vi "Step_Delay_Tommaso_fixed_EPICS2.vi"() -> ()   [LabVIEW 2020]
uses:
  <vilib>/DAQmx/write.llb/DAQmx Write (Analog DBL 1Chan 1Samp).vi
  <vilib>/DAQmx/miscellaneous.llb/DAQmx Fill In Error Info.vi
  <vilib>/DAQmx/create/channels.llb/DAQmx Create Channel (AO-Voltage-Basic).vi
  <userlib>/caLab/Private/Put_Boolean-1D_PV.vi
  <userlib>/caLab/Private/Put_DBL_PV.vi
  <vilib>/Analysis/1siggen.llb/Ramp Pattern by Delta.vi
  libs/Newport ESP301/Newport ESP301.lvlib
  <vilib>/Analysis/NI_AALBase.lvlib
panel:
  in  "WP2 pos B":dbl=30.0
  in  "WP1 pos B":dbl=10.0
  in  "WP2 pos A":dbl=35.0
  in  "WP1 pos A":dbl=15.0
  out "moving":bool
  out "running":bool
  out "wp2 position [deg]":dbl=35.0 format="%.6g"
  out "wp1 position [deg]":dbl=15.0 format="%.6g"
  in  "Tab Control":enum32{"equally spaced", "user-defined"}(tab)
  in  "StepSize [fs]":i32=1000
  out "StepSize [mm]":dbl=0.14989622900000002
  in  "Wait time [ms]":u32=1000
  in  "go2p1":bool
  in  "p2 [mm]":dbl=0.1
  in  "p1 [mm]":dbl=-0.1
  in  "Delta2 [fs]":dbl=6384.750346187828
  in  "Delta1 [fs]":dbl=5050.49396539522
  in  "Dwell_positions":string[][](table)=[["5000", "3000"], ["5100", "3000"], ["5200", "5000"], ["5300", "5000"], ["5500", "5000"], ["6000", "10000"], ["", ""], ["", ""]]
  out "IOC started":bool=TRUE
  in  "Config File":path=path "T:/trARPES/Labview/Front ends/METIS_delayscan/delayScanEPICS.conf" caption="Soft IOC configuration file"
  in  "Configuration Set":T1(array[cluster])=[{"PV name"="trARPES:DelayStage:t0", "description"="Delay Stage time zero Position", "data type"="ai", "number of elements (waveform only)"=1, "element size (waveform only)"="", []}, {"PV name"="trARPES:DelayStage:p1", "description"="Delay Stage range start", "data type"="ai", "number of elements (waveform only)"=1, "element size (waveform only)"="", []}, {"PV name"="trARPES:DelayStage:p2", "description"="Delay Stage range end", "data type"="ai", "number of elements (waveform only)"=1, "element size (waveform only)"="", []}, {"PV name"="trARPES:DelayStage:Pos", "description"="Current Delay Stage position", "data type"="ai", "number of elements (waveform only)"=1, "element size (waveform only)"="", []}]
  in  "stop 2":bool
  in  "Enable?":bool=TRUE
  out "a":waveform(dbl)(graph)={"t0"=timestamp(3680562352.257453 s since 1904-01-01), "dt"=1.0, "Y"=[0.04235]}
  out "Waveform Chart":dbl(graph)=6.694
  out "x*y":dbl=6.694
  in  "physical channels":tag="Dev1/ao1"
  out "DAC error":errorcluster
  out "ESP error":errorcluster
  in  "set_vel":bool
  in  "velocity [fs/s]":dbl=66.71281903963042
  in  "vel_mm":dbl=0.01 caption="velocity [mm/s]"
  out "meas. velocity":dbl
  out "output voltage":dbl=6.694
  in  "start":bool
  out "position [mm]":dbl=0.04235
  in  "interpolate output":bool
  in  "Reference [mm]":dbl=-0.85705
  in  "Axis (1)":i32[](array[numeric])=[3, 2, 1] min=1 max=3
  in  "Serial Link (RS232)":enum16{"RS232", "USB"}(ring)
  in  "VISA resource name":refnum<visa-resource-name>="COM8"
  in  "main_close":bool
  # "Interface panel"
  # "Velocity panel"
  # "delay"
  # "wp1"
  # "wp2"
  # "Positions panel"
  # "Measurement Mode"
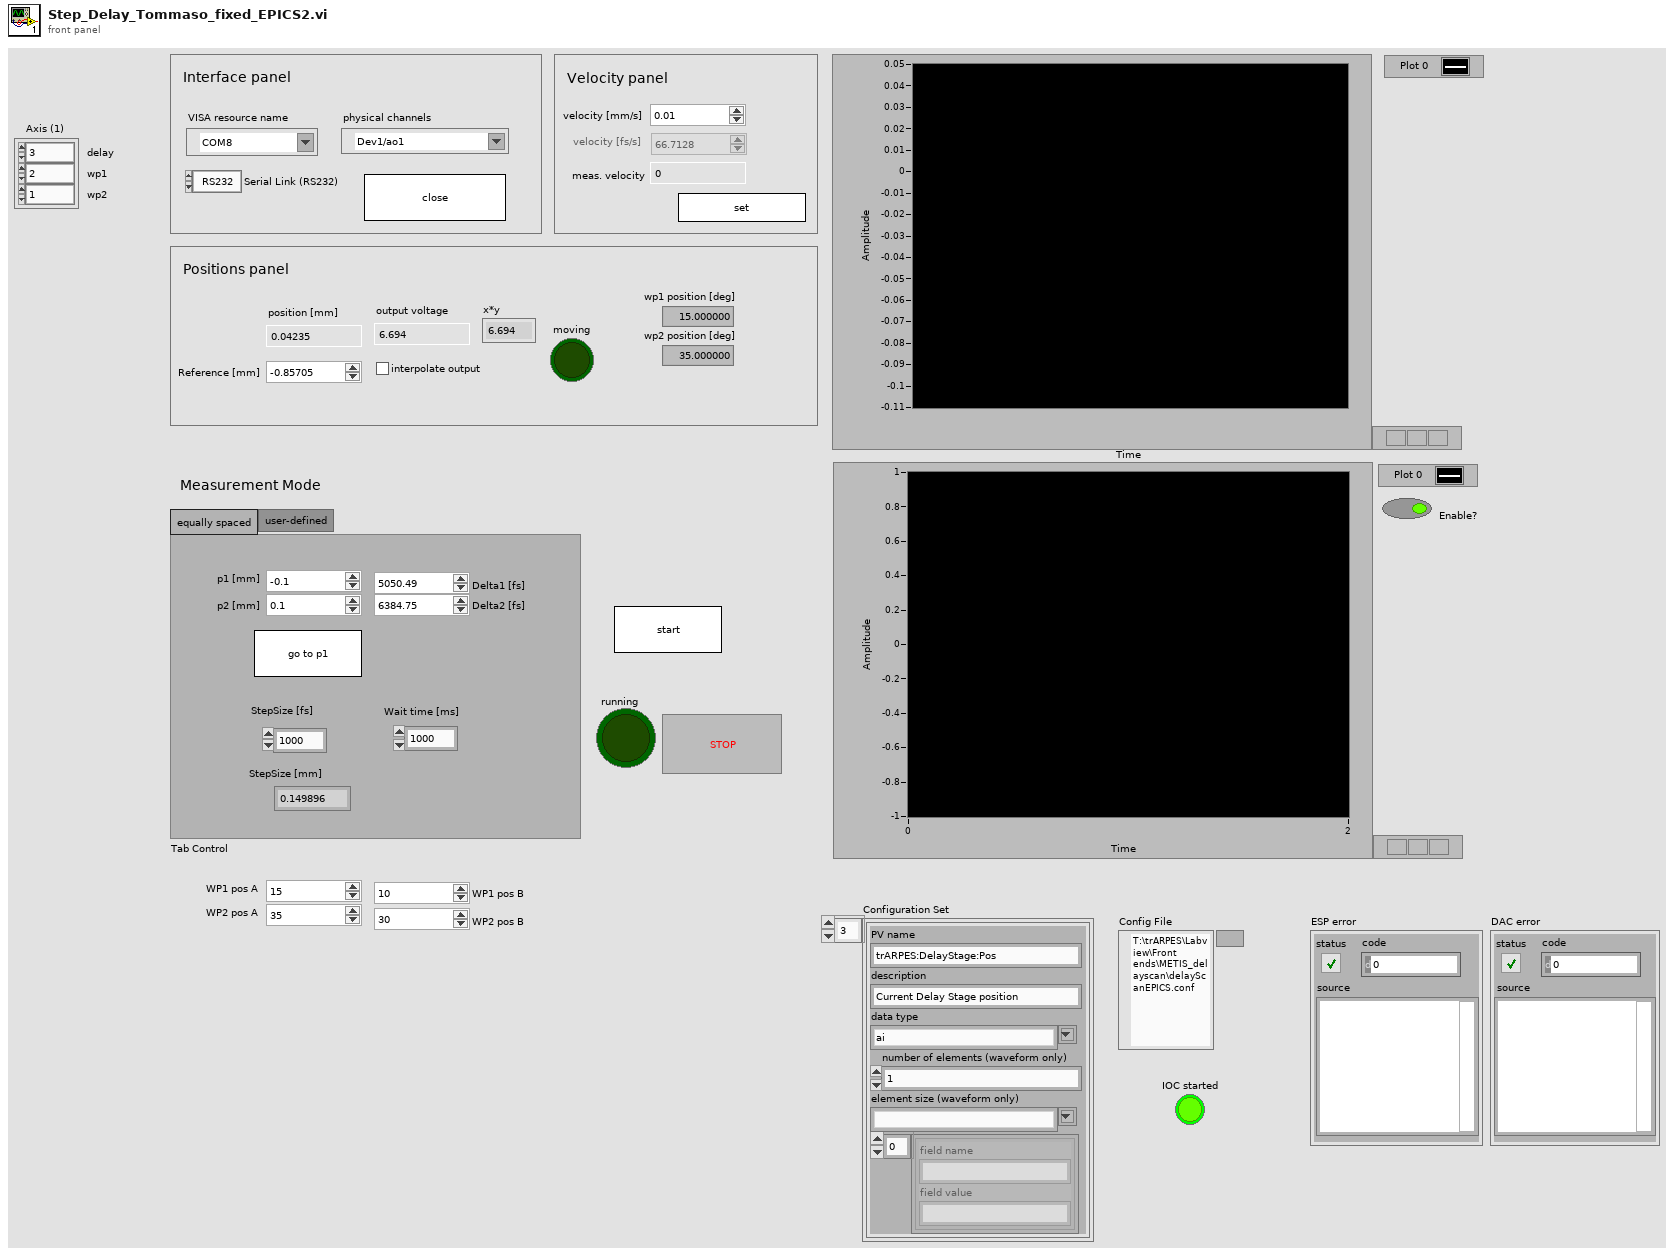
[diagram p1: front panel]
types:
  T1 = cluster{"PV name":string, "description":string, "data type":string, "number of elements (waveform only)":i32, "element size (waveform only)":string, cluster{"field name":string, "field value":string}[]}[]
  T2 = cluster{"dev1_data":refnum<queue>, "dev2_data":refnum<queue>}
  T3 = cluster{"dev1_cmd":refnum<queue>, "dev2_cmd":refnum<queue>, "meas_cmd":refnum<queue>}
  T4 = cluster{"PV Name":string, "Data Type":string, "Fields":cluster{"Field Name":string, "Field Value":string}[]}[]
  T5 = cluster{"PV Name":string, "Data Type":string, "Fields":cluster{"Field Name":string, "Field Value":string}[]}
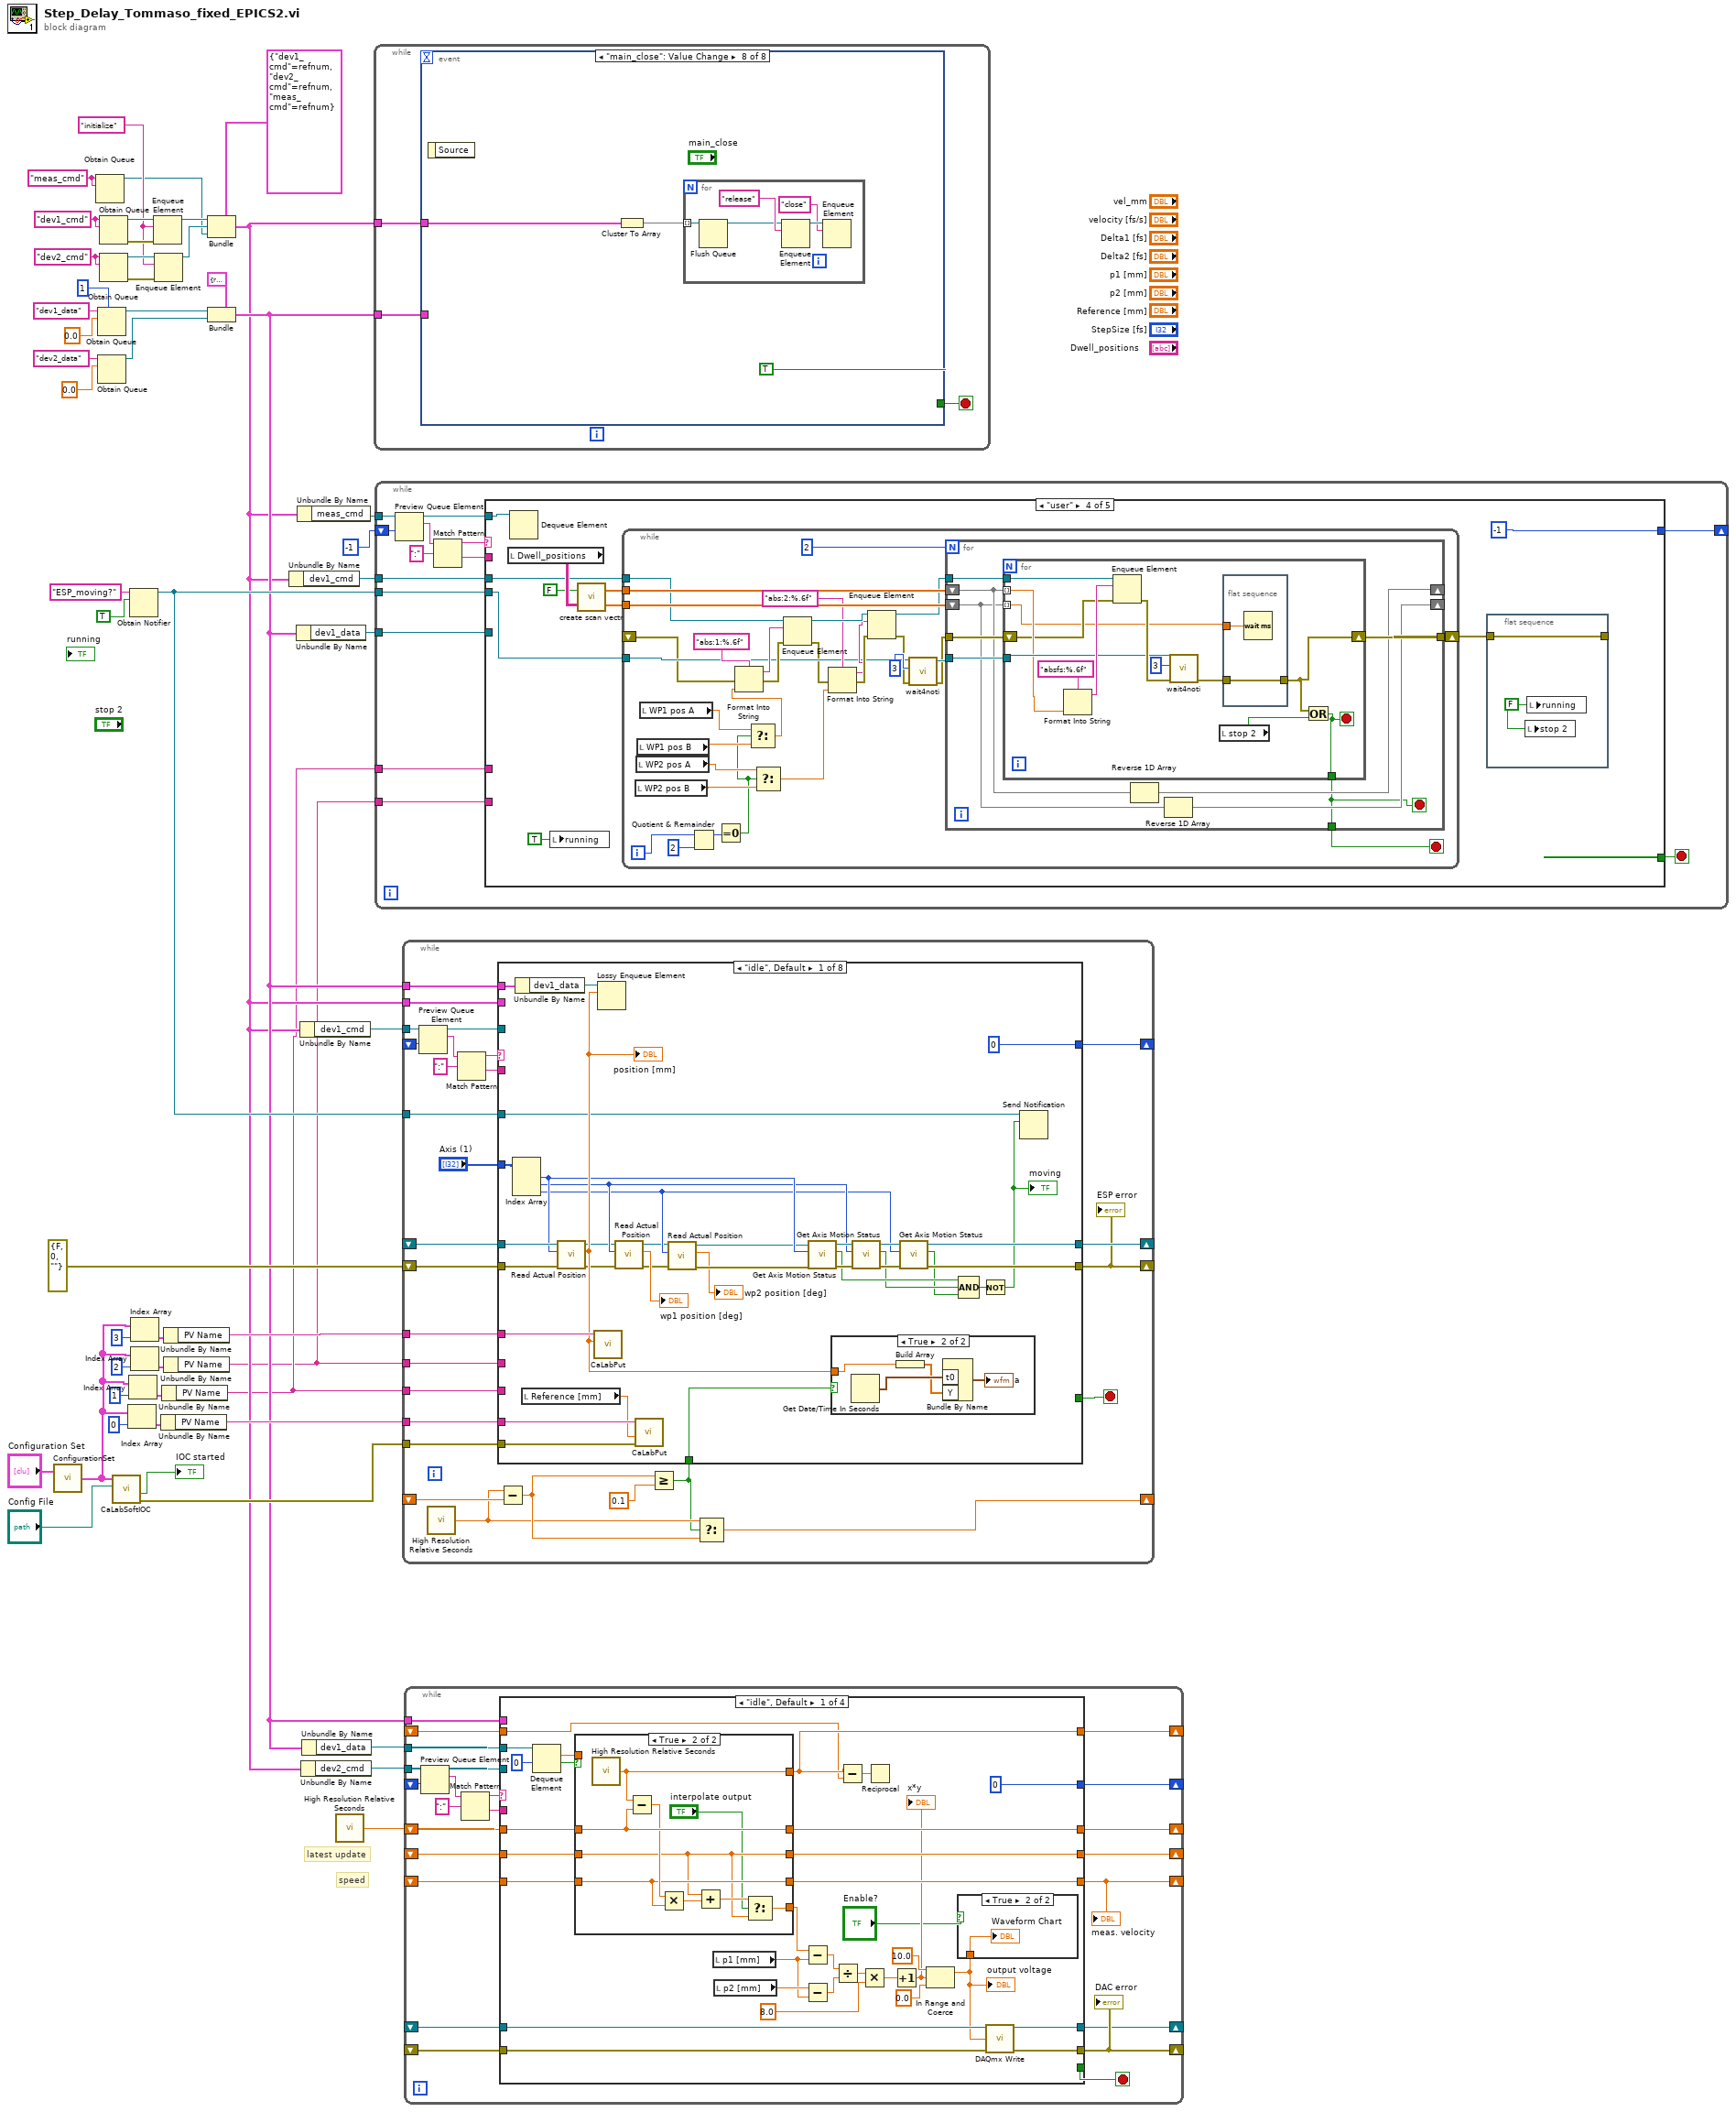
[diagram p0: block diagram]
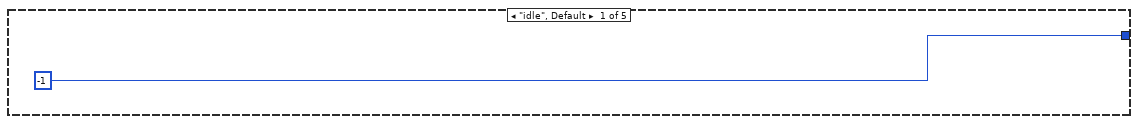
[diagram p2: hidden frame]
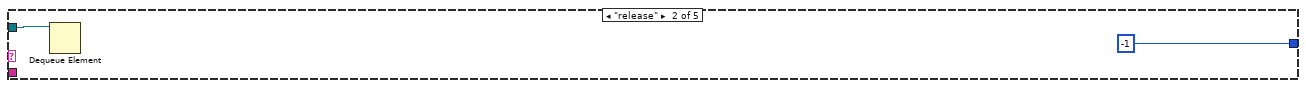
[diagram p3: hidden frame]
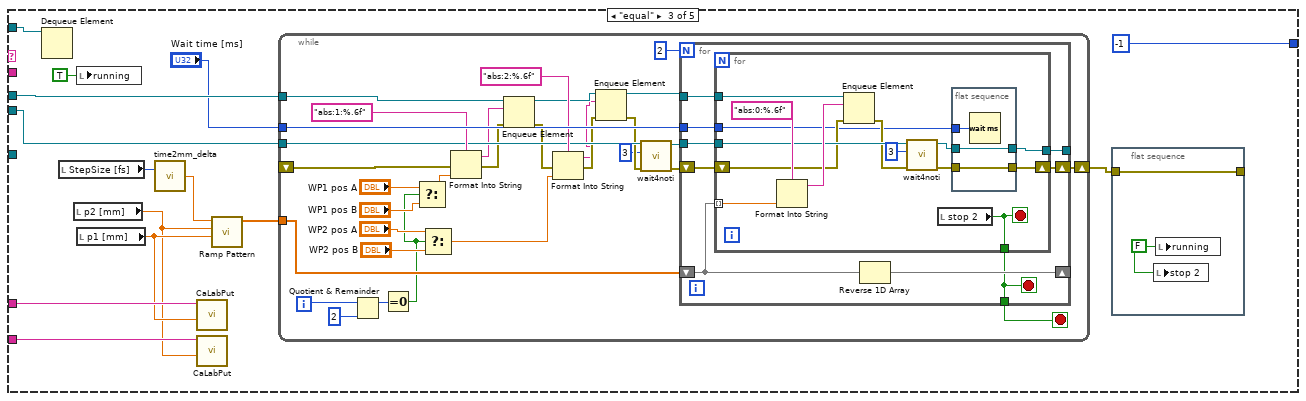
[diagram p4: hidden frame]
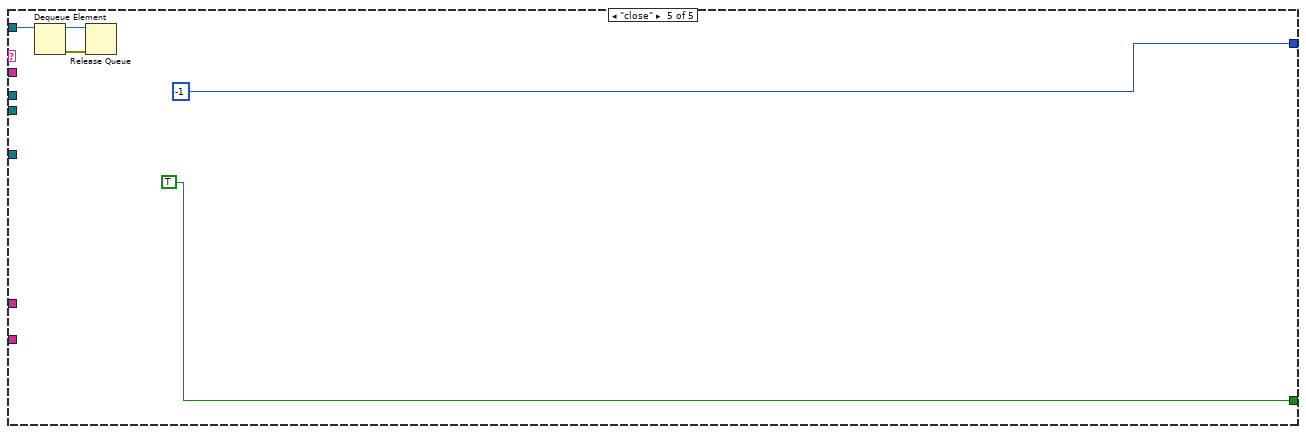
[diagram p5: hidden frame]
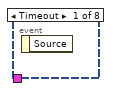
[diagram p6: hidden frame]
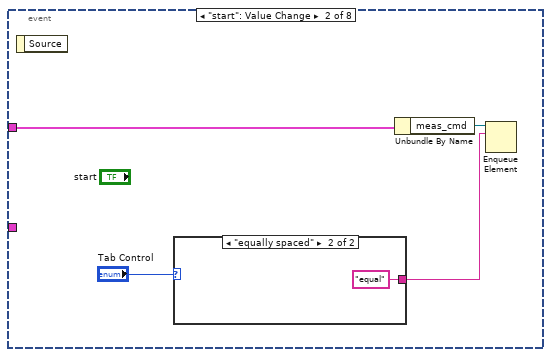
[diagram p7: hidden frame]
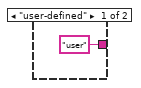
[diagram p8: hidden frame]
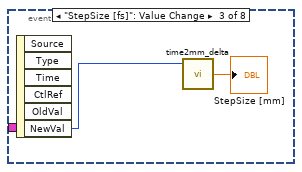
[diagram p9: hidden frame]
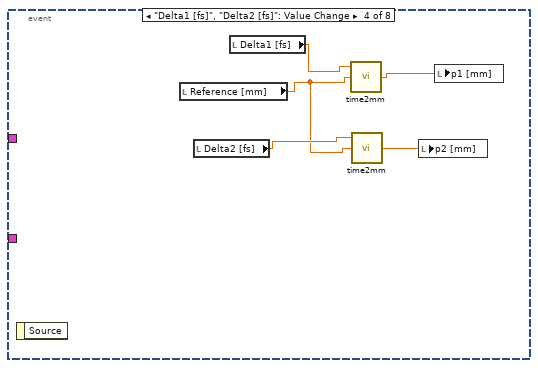
[diagram p10: hidden frame]
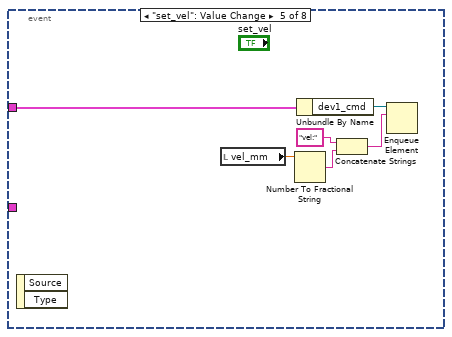
[diagram p11: hidden frame]
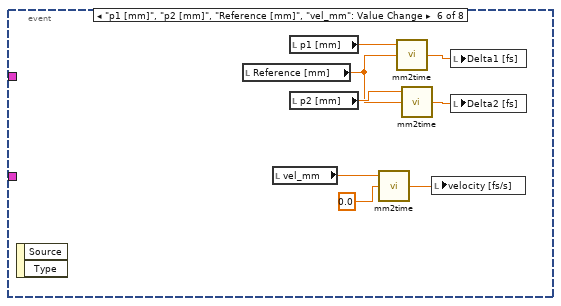
[diagram p12: hidden frame]
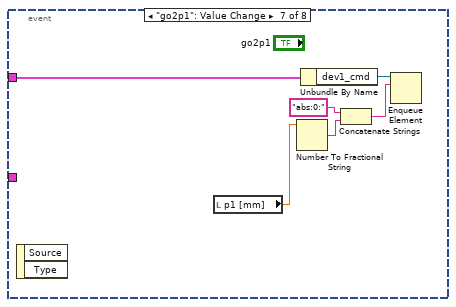
[diagram p13: hidden frame]
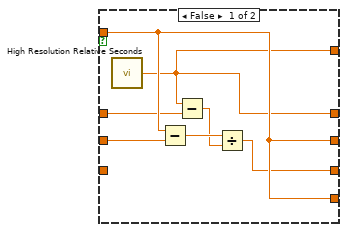
[diagram p15: hidden frame]
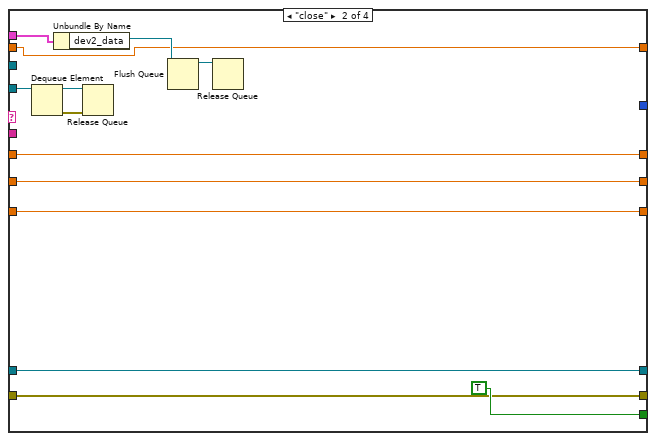
[diagram p16: hidden frame]
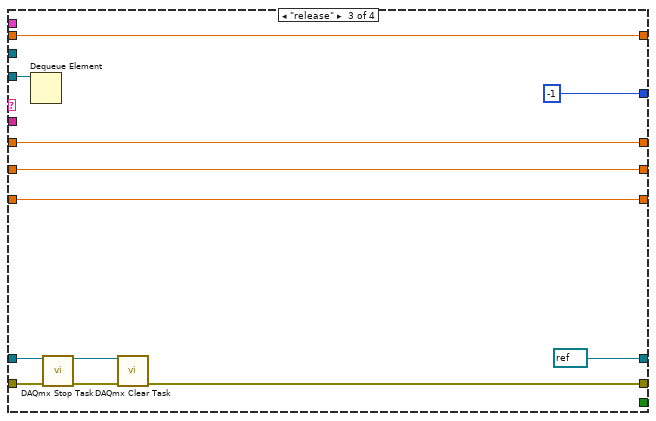
[diagram p17: hidden frame]
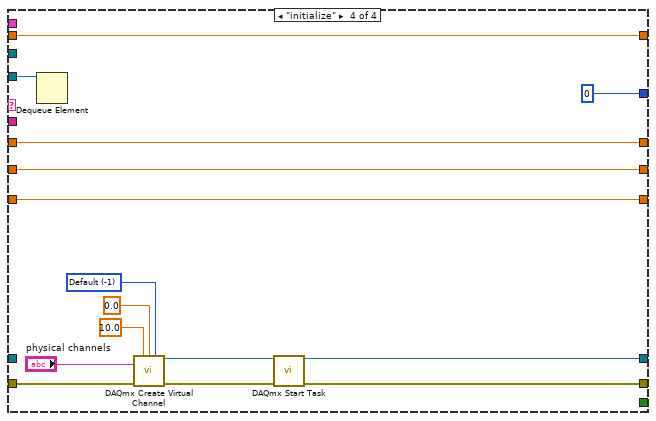
[diagram p18: hidden frame]
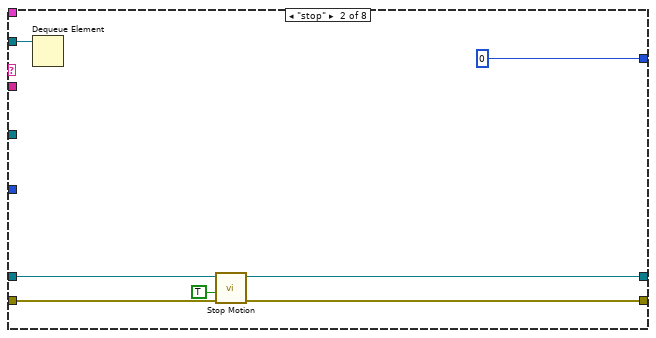
[diagram p20: hidden frame]
diagram:
  w12 = "meas_cmd" ("name (unnamed)")
  w39 = "dev2_cmd" ("name (unnamed)")
  w45 = "initialize" ("element")
  w40 = "dev1_cmd" ("name (unnamed)")
  # "speed"
  # "latest update"
  n1 = call <userlib>:"ConfigurationSet.vi"("Configuration Set"="Configuration Set") -> ("PV set"=w18:T4)  [unwired: 1 in]
  n2 = Obtain Queue(name (unnamed)=w12, element data type=w12) -> (queue out=w1:refnum<queue>)  [unwired: 3 in, 2 out]
  n3 = Obtain Queue(max queue size (-1, unlimited)=1, name (unnamed)="dev1_data", element data type=0.0) -> (queue out=w36:refnum<queue>)  [unwired: 2 in, 2 out]
  n4 = Obtain Queue(name (unnamed)="dev2_data", element data type=0.0) -> (queue out=w35:refnum<queue>)  [unwired: 3 in, 2 out]
  n5 = Obtain Queue(name (unnamed)=w40, element data type=w40) -> (queue out=w51:refnum<queue>, error out=w50:errorcluster)  [unwired: 3 in, 1 out]
  n6 = Obtain Queue(name (unnamed)=w39, element data type=w39) -> (queue out=w46:refnum<queue>, error out=w47:errorcluster)  [unwired: 3 in, 1 out]
  n7 = call <userlib>:"CaLabSoftIOC.vi"("Config File"="Config File", "PV set"=w18) -> ("error out"=w16:errorcluster, "IOC started"=→"IOC started":bool)  [unwired: 4 in, 2 out]
  n8 = Index Array(array=w18, index=0) -> (element=w27:T5)
  n9 = Index Array(array=w18, index=1) -> (element=w23:T5)
  n10 = Obtain Notifier(name (unnamed)="ESP_moving?", notification data type=TRUE) -> (notifier out=w9:refnum<notifier>)  [unwired: 2 in, 2 out]
  n11 = Index Array(array=w18, index=3) -> (element=w19:T5)
  n12 = Index Array(array=w18, index=2) -> (element=w22:T5)
  n13 = Enqueue Element(queue=w51, element=w45, error in (no error)=w50) -> (queue out=w48:refnum<queue>)  [unwired: 1 in, 2 out]
  n14 = Enqueue Element(queue=w46, element=w45, error in (no error)=w47) -> (queue out=w44:refnum<queue>)  [unwired: 1 in, 2 out]
  n15 = Unbundle By Name(w27) -> ("PV Name"=w15:string)
  n16 = Unbundle By Name(w23) -> ("PV Name"=w3:string)
  n17 = Unbundle By Name(w19) -> ("PV Name"=w14:string)
  n18 = Unbundle By Name(w22) -> ("PV Name"=w2:string)
  n19 = Bundle(cluster=T3 {"dev1_cmd"=refnum, "dev2_cmd"=refnum, "meas_cmd"=refnum}, "dev1_cmd"=w48, "dev2_cmd"=w44, "meas_cmd"=w1) -> (w5:T3)
  n20 = Bundle(cluster=T2 {"dev1_data"=refnum, "dev2_data"=refnum}, "dev1_data"=w36, "dev2_data"=w35) -> (w7:T2)
  n21 = Unbundle By Name(w5) -> ("dev1_cmd"=w4:refnum<queue>)
  n22 = Unbundle By Name(w7) -> ("dev1_data"=w6:refnum<queue>)
  n23 = Unbundle By Name(w5) -> ("meas_cmd"=w13:refnum<queue>)
  n24 = Unbundle By Name(w5) -> ("dev1_cmd"=w41:refnum<queue>)
  n25 = Unbundle By Name(w5) -> ("dev2_cmd"=w32:refnum<queue>)
  n26 = Unbundle By Name(w7) -> ("dev1_data"=w31:refnum<queue>)
  n27 = call <vilib>:"High Resolution Relative Seconds.vi"() -> ("relative seconds"=w30:dbl)
  n28 = while {
    tunnel: w5 -> [w54]
    tunnel: w7 -> [w53]
    stop <- w52 stop-if-true
    n29 = event shown="[7] \"main_close\": Value Change" {
      selector: _ -> [_ _ _ _ _ _ _ _]
      dyn-events: _ -> [_ _ _ _ _ _ _ _]
      timeout: _ -> [_ _ _ _ _ _ _ _]
      tunnel: w54 -> [_ w57 _ _ w69 _ w87 w90]
      tunnel: w53 -> [_ _ _ _ _ _ _ _]
      tunnel: [_ _ _ _ _ _ _ TRUE] -> w52
      event Timeout {
        n30 = event-data() -> ()  [unwired: 1 in, 1 out]
      }
      event "start": Value Change {
        n31 = event-data() -> ()  [unwired: 1 in, 1 out]
        n32 = case shown="\"equally spaced\"" "Tab Control" {
          tunnel: ["user" "equal"] -> w55
          frame "user-defined" {
          }
          frame "equally spaced" {
          }
        }
        n33 = Unbundle By Name(w57) -> ("meas_cmd"=w58:refnum<queue>)
        n34 = Enqueue Element(queue=w58, element=w55) -> ()  [unwired: 2 in, 3 out]
      }
      event "StepSize [fs]": Value Change {
        n35 = event-data() -> ("NewVal"=w61:i32)  [unwired: 1 in, 5 out]
        n36 = call "time2mm_delta.vi"("Delta time"=w61) -> ("Delta position (mm)"=→"StepSize [mm]":dbl)  [unwired: 2 in]
      }
      event "Delta1 [fs]", "Delta2 [fs]": Value Change {
        n37 = event-data() -> ()  [unwired: 1 in, 1 out]
        n38 = local read "Reference [mm]"() -> (w64:dbl)
        n39 = local read "Delta2 [fs]"() -> (w65:dbl)
        n40 = local read "Delta1 [fs]"() -> (w67:dbl)
        n41 = call "time2mm.vi"("Offset (mm)"=w64, "time"=w67) -> ("position (mm)"=w66:dbl)  [unwired: 1 in]
        n42 = call "time2mm.vi"("Offset (mm)"=w64, "time"=w65) -> ("position (mm)"=w63:dbl)  [unwired: 1 in]
        n43 = local write "p2 [mm]"(w63) -> ()
        n44 = local write "p1 [mm]"(w66) -> ()
      }
      event "set_vel": Value Change {
        n45 = event-data() -> ()  [unwired: 1 in, 2 out]
        n46 = local read "vel_mm"() -> (w68:dbl)
        n47 = Number To Fractional String(number=w68) -> (F-format string=w72:string)  [unwired: 3 in]
        n48 = Unbundle By Name(w69) -> ("dev1_cmd"=w73:refnum<queue>)
        n49 = Concatenate Strings("vel:" ("string"), w72) -> (w71:string)
        n50 = Enqueue Element(queue=w73, element=w71) -> ()  [unwired: 2 in, 3 out]
      }
      event "p1 [mm]", "p2 [mm]", "Reference [mm]", "vel_mm": Value Change {
        n51 = event-data() -> ()  [unwired: 1 in, 2 out]
        n52 = local read "Reference [mm]"() -> (w79:dbl)
        n53 = local read "vel_mm"() -> (w76:dbl)
        n54 = local read "p1 [mm]"() -> (w80:dbl)
        n55 = local read "p2 [mm]"() -> (w81:dbl)
        n56 = call "mm2time.vi"("Offset (mm)"=0.0, "distance (mm)"=w76) -> ("time in fs"=w75:dbl)  [unwired: 1 in]
        n57 = call "mm2time.vi"("Offset (mm)"=w79, "distance (mm)"=w80) -> ("time in fs"=w77:dbl)  [unwired: 1 in]
        n58 = call "mm2time.vi"("Offset (mm)"=w79, "distance (mm)"=w81) -> ("time in fs"=w78:dbl)  [unwired: 1 in]
        n59 = local write "velocity [fs/s]"(w75) -> ()
        n60 = local write "Delta1 [fs]"(w77) -> ()
        n61 = local write "Delta2 [fs]"(w78) -> ()
      }
      event "go2p1": Value Change {
        n62 = event-data() -> ()  [unwired: 1 in, 2 out]
        n63 = local read "p1 [mm]"() -> (w82:dbl)
        n64 = Number To Fractional String(number=w82) -> (F-format string=w85:string)  [unwired: 3 in]
        n65 = Unbundle By Name(w87) -> ("dev1_cmd"=w86:refnum<queue>)
        n66 = Concatenate Strings("abs:0:" ("string"), w85) -> (w83:string)
        n67 = Enqueue Element(queue=w86, element=w83) -> ()  [unwired: 2 in, 3 out]
      }
      event "main_close": Value Change {
        n68 = event-data() -> ()  [unwired: 1 in, 1 out]
        n69 = Cluster To Array(cluster=w90) -> (array=w89:refnum<queue>[])
        n70 = for {
          tunnel: w89 -> [w95] mode=indexing
          n71 = Flush Queue(queue=w95) -> (queue out=w91:refnum<queue>)  [unwired: 1 in, 2 out]
          n72 = Enqueue Element(queue=w91, element="release") -> (queue out=w93:refnum<queue>)  [unwired: 2 in, 2 out]
          n73 = Enqueue Element(queue=w93, element="close") -> ()  [unwired: 2 in, 3 out]
        }
      }
    }
  }
  n74 = while {
    tunnel: w13 -> [w108]
    tunnel: w9 -> [w102]
    shift-right: [w100] -> _
    shift-left: -1 -> [w101]
    tunnel: w6 -> [w99]
    tunnel: w4 -> [w98]
    tunnel: w3 -> [w97]
    tunnel: w2 -> [w96]
    stop <- w104 stop-if-true
    n75 = Preview Queue Element(queue=w108, timeout in ms (-1)=w101) -> (queue out=w103:refnum<queue>, element=w107:string)  [unwired: 1 in, 2 out]
    n76 = Match Pattern(string=w107, regular expression=":") -> (before substring=w106:string, after substring=w105:string)  [unwired: 1 in, 2 out]
    n77 = case shown="\"user\"" w106 {
      tunnel: w105 -> [_ _ _ _ _]
      tunnel: [_ _ _ _ TRUE] -> w104
      tunnel: w103 -> [_ w112 w115 w190 w255]
      tunnel: w102 -> [_ _ w123 w192 _]
      tunnel: [-1 -1 -1 -1 -1] -> w100
      tunnel: w99 -> [_ _ _ _ _]
      tunnel: w98 -> [_ _ w124 w193 _]
      tunnel: w97 -> [_ _ w122 _ _]
      tunnel: w96 -> [_ _ w120 _ _]
      frame "idle", Default {
      }
      frame "release" {
        n78 = Dequeue Element(queue=w112) -> ()  [unwired: 2 in, 4 out]
      }
      frame "equal" {
        n79 = Dequeue Element(queue=w115) -> ()  [unwired: 2 in, 4 out]
        n80 = local read "StepSize [fs]"() -> (w126:i32)
        n81 = local read "p2 [mm]"() -> (w119:dbl)
        n82 = local write "running"(TRUE ("running")) -> ()
        n83 = local read "p1 [mm]"() -> (w121:dbl)
        n84 = call "time2mm_delta.vi"("Delta time"=w126) -> ("Delta position (mm)"=w125:dbl)  [unwired: 2 in]
        n85 = call-poly <userlib>:"CaLabPut.vi"("Timeout (3)"=w121, "PV Name"=w122) -> ()  [unwired: 6 in, 4 out]
        n86 = call-poly <userlib>:"CaLabPut.vi"("Timeout (3)"=w119, "PV Name"=w120) -> ()  [unwired: 6 in, 4 out]
        n87 = call-poly <vilib>:"Ramp Pattern.vi"("start"=w121, "end"=w119, "delta"=w125) -> ("Ramp Pattern"=w117:dbl[])  [unwired: 6 in, 2 out]
        n88 = while {
          tunnel: w117 -> [w155]
          tunnel: w124 -> [w137]
          tunnel: w123 -> [w150]
          tunnel: "Wait time [ms]" -> [w158]
          shift-right: [w157] -> w114
          shift-left: _ -> [w152]
          i -> [w148]
          stop <- w159 stop-if-true
          n89 = Quotient & Remainder(x=w148, y=2) -> (x-y*floor(x/y)=w146:i32)  [unwired: 1 out]
          n90 = Equal To 0?(x=w146) -> (x = 0?=w139:bool)
          n91 = Select(t="WP1 pos A", s=w139, f="WP1 pos B") -> (s? t:f=w141:dbl)
          n92 = Select(t="WP2 pos A", s=w139, f="WP2 pos B") -> (s? t:f=w140:dbl)
          n93 = Format Into String(format string="abs:1:%.6f", error in=w152, w141) -> (resulting string=w138:string, error out=w136:errorcluster)  [unwired: 1 in]
          n94 = Enqueue Element(queue=w137, element=w138, error in (no error)=w136) -> (queue out=w133:refnum<queue>, error out=w135:errorcluster)  [unwired: 1 in, 1 out]
          n95 = Format Into String(format string="abs:2:%.6f", error in=w135, w140) -> (resulting string=w130:string, error out=w132:errorcluster)  [unwired: 1 in]
          n96 = Enqueue Element(queue=w133, element=w130, error in (no error)=w132) -> (queue out=w134:refnum<queue>, error out=w131:errorcluster)  [unwired: 1 in, 1 out]
          n97 = call "wait4noti.vi"("error in (no error)"=w131, "N"=3, "notifier"=w150) -> ("error out"=w151:errorcluster, "notifier out"=w149:refnum<notifier>)  [unwired: 7 in]
          n98 = for {
            N: 2 -> [_]
            tunnel: w134 -> [w168]
            tunnel: w149 -> [w167]
            tunnel: [w161] -> w159
            tunnel: w158 -> [w166]
            shift-right: [w163] -> _
            shift-left: w155 -> [w162]
            tunnel: [w160] -> _
            shift-right: [w165] -> w157
            shift-left: w151 -> [w164]
            stop <- w161 stop-if-true
            n99 = for {
              tunnel: w162 -> [w180] mode=indexing
              tunnel: w168 -> [w182]
              tunnel: w167 -> [w178]
              tunnel: [w176] -> w161
              tunnel: w166 -> [w172]
              shift-right: [w175] -> w165
              shift-left: w164 -> [w173]
              tunnel: [w171] -> w160
              stop <- w176 stop-if-true
              n100 = Format Into String(format string="abs:0:%.6f", w180) -> (resulting string=w179:string)  [unwired: 2 in, 1 out]
              n101 = Enqueue Element(queue=w182, element=w179, error in (no error)=w173) -> (error out=w177:errorcluster)  [unwired: 1 in, 2 out]
              n102 = call "wait4noti.vi"("error in (no error)"=w177, "N"=3, "notifier"=w178) -> ("error out"=w174:errorcluster, "notifier out"=w170:refnum<notifier>)  [unwired: 7 in]
              n103 = local read "stop 2"() -> (w176:bool)
              n104 = flat-sequence {
                tunnel: [w185] -> w175
                tunnel: w174 -> [w185]
                tunnel: w172 -> [w184]
                tunnel: [w183] -> w171
                tunnel: w170 -> [w183]
                frame #0 {
                  n105 = Wait (ms)(milliseconds to wait=w184) -> ()  [unwired: 1 out]
                }
              }
            }
            n106 = Reverse 1D Array(array=w162) -> (reversed array=w163:dbl[])
          }
        }
        n107 = flat-sequence {
          tunnel: w114 -> [w127]
          tunnel: [w127] -> _
          frame #0 {
            w128 = FALSE ("running")
            n108 = local write "stop 2"(w128) -> ()
            n109 = local write "running"(w128) -> ()
          }
        }
      }
      frame "user" {
        n110 = local read "Dwell_positions"() -> (w195:string[][])
        n111 = Dequeue Element(queue=w190) -> ()  [unwired: 2 in, 4 out]
        n112 = local write "running"(TRUE ("running")) -> ()
        n113 = call "create scan vectr.vi"("Table Control"=w195, "waypoint mode?"=FALSE) -> ("Array 2"=w188:dbl[], "Array"=w189:dbl[])
        n114 = while {
          tunnel: w193 -> [w213]
          tunnel: w192 -> [w215]
          tunnel: w188 -> [w224]
          shift-right: [w227] -> w187
          shift-left: _ -> [w208]
          tunnel: w189 -> [w225]
          i -> [w206]
          stop <- w228 stop-if-true
          n115 = local read "WP2 pos B"() -> (w202:dbl)
          n116 = local read "WP2 pos A"() -> (w203:dbl)
          n117 = local read "WP1 pos B"() -> (w204:dbl)
          n118 = local read "WP1 pos A"() -> (w205:dbl)
          n119 = Quotient & Remainder(x=w206, y=2) -> (x-y*floor(x/y)=w201:i32)  [unwired: 1 out]
          n120 = Equal To 0?(x=w201) -> (x = 0?=w200:bool)
          n121 = Select(t=w205, s=w200, f=w204) -> (s? t:f=w199:dbl)
          n122 = Format Into String(format string="abs:1:%.6f", error in=w208, w199) -> (resulting string=w223:string, error out=w222:errorcluster)  [unwired: 1 in]
          n123 = Select(t=w203, s=w200, f=w202) -> (s? t:f=w198:dbl)
          n124 = Enqueue Element(queue=w213, element=w223, error in (no error)=w222) -> (queue out=w221:refnum<queue>, error out=w209:errorcluster)  [unwired: 1 in, 1 out]
          n125 = Format Into String(format string="abs:2:%.6f", error in=w209, w198) -> (resulting string=w219:string, error out=w220:errorcluster)  [unwired: 1 in]
          n126 = Enqueue Element(queue=w221, element=w219, error in (no error)=w220) -> (queue out=w212:refnum<queue>, error out=w210:errorcluster)  [unwired: 1 in, 1 out]
          n127 = call "wait4noti.vi"("error in (no error)"=w210, "N"=3, "notifier"=w215) -> ("error out"=w211:errorcluster, "notifier out"=w214:refnum<notifier>)  [unwired: 7 in]
          n128 = for {
            N: 2 -> [_]
            tunnel: w212 -> [w237]
            tunnel: w214 -> [w236]
            tunnel: [w229] -> w228
            tunnel: w211 -> [w235]
            tunnel: [w234] -> w227
            shift-right: [w231] -> _
            shift-left: w225 -> [w233]
            shift-right: [w230] -> _
            shift-left: w224 -> [w232]
            stop <- w229 stop-if-true
            n129 = for {
              tunnel: w233 -> [w245] mode=indexing
              tunnel: w237 -> [w247]
              tunnel: w236 -> [w246]
              tunnel: [w240] -> w229
              tunnel: w232 -> [w239] mode=indexing
              shift-right: [w241] -> w234
              shift-left: w235 -> [w244]
              stop <- w240 stop-if-true
              n130 = Format Into String(format string="absfs:%.6f", w245) -> (resulting string=w250:string)  [unwired: 2 in, 1 out]
              n131 = Enqueue Element(queue=w247, element=w250, error in (no error)=w244) -> (error out=w249:errorcluster)  [unwired: 1 in, 2 out]
              n132 = call "wait4noti.vi"("error in (no error)"=w249, "N"=3, "notifier"=w246) -> ("error out"=w243:errorcluster)  [unwired: 7 in, 1 out]
              n133 = local read "stop 2"() -> (w242:bool)
              n134 = flat-sequence {
                tunnel: [w252] -> w241
                tunnel: w243 -> [w252]
                tunnel: w239 -> [w251]
                frame #0 {
                  n135 = Wait (ms)(milliseconds to wait=w251) -> ()  [unwired: 1 out]
                }
              }
              n136 = Or(x=w241, y=w242) -> (x .or. y?=w240:bool)
            }
            n137 = Reverse 1D Array(array=w233) -> (reversed array=w231:dbl[])
            n138 = Reverse 1D Array(array=w232) -> (reversed array=w230:dbl[])
          }
        }
        n139 = flat-sequence {
          tunnel: w187 -> [w196]
          tunnel: [w196] -> _
          frame #0 {
            w197 = FALSE ("running")
            n140 = local write "stop 2"(w197) -> ()
            n141 = local write "running"(w197) -> ()
          }
        }
      }
      frame "close" {
        n142 = Dequeue Element(queue=w255) -> (queue out=w254:refnum<queue>, error out=w256:errorcluster)  [unwired: 2 in, 2 out]
        n143 = Release Queue(queue=w254, error in (no error)=w256) -> ()  [unwired: 1 in, 3 out]
      }
    }
  }
  n144 = while {
    tunnel: w5 -> [w280]
    tunnel: w41 -> [w285]
    tunnel: w7 -> [w277]
    shift-right: [w275] -> _
    shift-left: _ -> [w276]
    shift-right: [w274] -> _
    shift-left: _ -> [w271]
    shift-right: [w273] -> _
    shift-left: errorcluster {"status"=FALSE, "code"=0, "source"=""} ("error out") -> [w272]
    shift-right: [w264] -> _
    shift-left: _ -> [w269]
    tunnel: w16 -> [w263]
    tunnel: w15 -> [w262]
    tunnel: w3 -> [w261]
    tunnel: w2 -> [w260]
    tunnel: w14 -> [w259]
    tunnel: w9 -> [w258]
    stop <- w278 stop-if-true
    n145 = Preview Queue Element(queue=w285, timeout in ms (-1)=w276) -> (queue out=w279:refnum<queue>, element=w284:string)  [unwired: 1 in, 2 out]
    n146 = call <vilib>:"High Resolution Relative Seconds.vi"() -> ("relative seconds"=w266:dbl)
    n147 = Match Pattern(string=w284, regular expression=":") -> (before substring=w282:string, after substring=w281:string)  [unwired: 1 in, 2 out]
    n148 = Subtract(x=w266, y=w269) -> (x-y=w267:dbl)
    n149 = Greater Or Equal?(x=w267, y=0.1) -> (x >= y?=w265:bool)
    n150 = case shown="\"idle\", Default" w282 {
      tunnel: w281 -> [_ _ w336 w354 w361 _ _ _]
      tunnel: w280 -> [_ _ _ _ _ _ _ _]
      tunnel: w279 -> [_ w326 w343 w355 w359 w375 w383 w393]
      tunnel: [_ _ _ _ _ TRUE _ _] -> w278
      tunnel: w277 -> [w319 _ _ _ _ w368 _ _]
      tunnel: [0 0 0 0 0 0 -1 0] -> w275
      tunnel: [w304 w329 w340 w348 w365 w371 refnum<visa-resource-name> refnum ("VISA resource name out") w390] -> w274
      tunnel: [w303 w328 w339 w347 w364 w370 w382 w389] -> w273
      tunnel: w272 -> [w316 w330 w341 w350 w363 w370 w380 _]
      tunnel: w271 -> [w317 w331 w342 w351 w362 w371 w377 _]
      tunnel: "Axis (1)" -> [w308 _ w337 w345 w357 _ _ w386]
      tunnel: w265 -> [w315 _ _ _ _ _ _ _]
      tunnel: w263 -> [w313 _ _ _ _ _ _ _]
      tunnel: w262 -> [w314 _ _ _ _ _ _ _]
      tunnel: w261 -> [_ _ _ _ _ _ _ _]
      tunnel: w260 -> [_ _ _ _ _ _ _ _]
      tunnel: w259 -> [w311 _ _ _ _ _ _ _]
      tunnel: w258 -> [w309 _ _ _ _ _ _ _]
      frame "idle", Default {
        n151 = Index Array(array=w308) -> (element #1=w307:i32, element #2=w300:i32, element #3=w299:i32)  [unwired: 3 in]
        n152 = Unbundle By Name(w319) -> ("dev1_data"=w318:refnum<queue>)
        n153 = local read "Reference [mm]"() -> (w312:dbl)
        n154 = call "Read Actual Position.vi"("error in (no error)"=w316, "Axis (1)"=w307, "VISA resource name"=w317) -> ("error out"=w294:errorcluster, "Position (units)"=w310:dbl, "VISA resource name out"=w298:refnum<visa-resource-name>)  [unwired: 2 in]
        "position [mm]" <- w310
        n155 = call-poly <userlib>:"CaLabPut.vi"("Value"=w310, "PV Name"=w311) -> ()  [unwired: 6 in, 4 out]
        n156 = Lossy Enqueue Element(queue=w318, element=w310) -> ()  [unwired: 1 in, 4 out]
        n157 = call "Read Actual Position.vi"("error in (no error)"=w294, "Axis (1)"=w300, "VISA resource name"=w298) -> ("error out"=w293:errorcluster, "Position (units)"=→"wp1 position [deg]":dbl, "VISA resource name out"=w297:refnum<visa-resource-name>)  [unwired: 2 in]
        n158 = call-poly <userlib>:"CaLabPut.vi"("Error in (no error)"=w313, "Timeout (3)"=w312, "PV Name"=w314) -> ()  [unwired: 5 in, 4 out]
        n159 = call "Read Actual Position.vi"("error in (no error)"=w293, "Axis (1)"=w299, "VISA resource name"=w297) -> ("error out"=w292:errorcluster, "Position (units)"=→"wp2 position [deg]":dbl, "VISA resource name out"=w296:refnum<visa-resource-name>)  [unwired: 2 in]
        n160 = call "Get Axis Motion Status.vi"("error in (no error)"=w292, "Axis (1)"=w307, "VISA resource name"=w296) -> ("error out"=w302:errorcluster, "Motion Done"=w290:bool, "VISA resource name out"=w306:refnum<visa-resource-name>)  [unwired: 2 in]
        n161 = case shown="True" w315 {
          tunnel: w310 -> [_ w324]
          frame False {
          }
          frame True {
            n162 = Get Date/Time In Seconds() -> (seconds since 1Jan1904=w323:timestamp)
            n163 = Build Array(w324) -> (w322:dbl[])
            n164 = Bundle By Name("t0"=w323, "Y"=w322) -> (→"a":waveform(dbl))  [unwired: 1 in]
          }
        }
        n165 = call "Get Axis Motion Status.vi"("error in (no error)"=w302, "Axis (1)"=w300, "VISA resource name"=w306) -> ("error out"=w301:errorcluster, "Motion Done"=w289:bool, "VISA resource name out"=w305:refnum<visa-resource-name>)  [unwired: 2 in]
        n166 = call "Get Axis Motion Status.vi"("error in (no error)"=w301, "Axis (1)"=w299, "VISA resource name"=w305) -> ("error out"=w303:errorcluster, "Motion Done"=w288:bool, "VISA resource name out"=w304:refnum<visa-resource-name>)  [unwired: 2 in]
        n167 = Compound Arithmetic op=AND(w290, w289, w288) -> (w287:bool)
        n168 = Not(x=w287) -> (.not. x?=w286:bool)
        "moving" <- w286
        n169 = Send Notification(notification=w286, notifier=w309) -> ()  [unwired: 1 in, 2 out]
      }
      frame "stop" {
        n170 = Dequeue Element(queue=w326) -> ()  [unwired: 2 in, 4 out]
        n171 = call "Stop Motion.vi"("error in (no error)"=w330, "Stop all axes (F)"=TRUE, "VISA resource name"=w331) -> ("error out"=w328:errorcluster, "VISA resource name out"=w329:refnum<visa-resource-name>)  [unwired: 3 in]
      }
      frame "abs" {
        n172 = Dequeue Element(queue=w343) -> ()  [unwired: 2 in, 4 out]
        n173 = Scan From String(format string="%u:%f", input string=w336) -> (output 1=w334:u32, output 2=w333:dbl)  [unwired: 4 in, 3 out]
        n174 = Index Array(array=w337, index=w334) -> (element=w332:i32)
        n175 = call "Move Absolute.vi"("error in (no error)"=w341, "Position (0 units)"=w333, "Axis (1)"=w332, "VISA resource name"=w342) -> ("error out"=w339:errorcluster, "VISA resource name out"=w340:refnum<visa-resource-name>)  [unwired: 2 in]
      }
      frame "absfs" {
        n176 = Index Array(array=w345) -> (element=w344:i32)  [unwired: 1 in]
        n177 = Dequeue Element(queue=w355) -> ()  [unwired: 2 in, 4 out]
        n178 = local read "Reference [mm]"() -> (w353:dbl)
        n179 = Fract/Exp String To Number(string=w354) -> (number=w352:dbl)  [unwired: 3 in, 1 out]
        n180 = call "time2mm.vi"("Offset (mm)"=w353, "time"=w352) -> ("position (mm)"=w349:dbl)  [unwired: 1 in]
        n181 = call "Move Absolute.vi"("error in (no error)"=w350, "Position (0 units)"=w349, "Axis (1)"=w344, "VISA resource name"=w351) -> ("error out"=w347:errorcluster, "VISA resource name out"=w348:refnum<visa-resource-name>)  [unwired: 2 in]
      }
      frame "vel" {
        n182 = Index Array(array=w357) -> (element=w356:i32)  [unwired: 1 in]
        n183 = Dequeue Element(queue=w359) -> ()  [unwired: 2 in, 4 out]
        n184 = Fract/Exp String To Number(string=w361) -> (number=w360:dbl)  [unwired: 3 in, 1 out]
        n185 = call "Set Velocity.vi"("error in (no error)"=w363, "Velocity (units/s)"=w360, "Axis (1)"=w356, "VISA resource name"=w362) -> ("error out"=w364:errorcluster, "VISA resource name out"=w365:refnum<visa-resource-name>)  [unwired: 2 in]
      }
      frame "close" {
        n186 = Dequeue Element(queue=w375) -> (queue out=w374:refnum<queue>, error out=w373:errorcluster)  [unwired: 2 in, 2 out]
        n187 = Unbundle By Name(w368) -> ("dev1_data"=w366:refnum<queue>)
        n188 = Release Queue(queue=w374, error in (no error)=w373) -> ()  [unwired: 1 in, 3 out]
        n189 = Flush Queue(queue=w366) -> (queue out=w367:refnum<queue>)  [unwired: 1 in, 2 out]
        n190 = Release Queue(queue=w367) -> ()  [unwired: 2 in, 3 out]
      }
      frame "release" {
        n191 = Dequeue Element(queue=w383) -> ()  [unwired: 2 in, 4 out]
        n192 = call "Stop Motion.vi"("error in (no error)"=w380, "Stop all axes (F)"=TRUE, "VISA resource name"=w377) -> ("error out"=w379:errorcluster, "VISA resource name out"=w378:refnum<visa-resource-name>)  [unwired: 3 in]
        n193 = call "Close.vi"("error in (no error)"=w379, "VISA resource name"=w378) -> ("error out"=w382:errorcluster)  [unwired: 9 in]
      }
      frame "initialize" {
        n194 = Dequeue Element(queue=w393) -> ()  [unwired: 2 in, 4 out]
        n195 = Index Array(array=w386) -> (element=w385:i32)  [unwired: 1 in]
        n196 = call "Initialize.vi"("VISA resource name"="VISA resource name", "error in (no error)"=errorcluster {"status"=FALSE, "code"=0, "source"=""}, "Serial Link (RS232)"="Serial Link (RS232)") -> ("VISA resource name out"=w392:refnum<visa-resource-name>, "error out"=w391:errorcluster)  [unwired: 6 in]
        n197 = call "Get Velocity.vi"("error in (no error)"=w391, "Axis (1)"=w385, "VISA resource name"=w392) -> ("error out"=w389:errorcluster, "Velocity (units/s)"=w388:dbl, "VISA resource name out"=w390:refnum<visa-resource-name>)  [unwired: 2 in]
        n198 = local write "vel_mm"(w388) -> ()
      }
    }
    "ESP error" <- w273
    n199 = Select(t=w266, s=w265, f=w267) -> (s? t:f=w264:dbl)
  }
  n200 = while {
    shift-right: [w412] -> _
    shift-left: _ -> [w413]
    shift-right: [w411] -> _
    shift-left: _ -> [w410]
    tunnel: w32 -> [w409]
    shift-right: [w408] -> _
    shift-left: _ -> [w407]
    tunnel: w31 -> [w406]
    shift-right: [w405] -> _
    shift-left: _ -> [w402]
    shift-right: [w404] -> _
    shift-left: w30 -> [w403]
    shift-right: [w397] -> _
    shift-left: _ -> [w401]
    tunnel: w7 -> [w400]
    shift-right: [w399] -> _
    shift-left: _ -> [w398]
    stop <- w414 stop-if-true
    n201 = Preview Queue Element(queue=w409, timeout in ms (-1)=w413) -> (queue out=w415:refnum<queue>, element=w419:string)  [unwired: 1 in, 2 out]
    n202 = Match Pattern(string=w419, regular expression=":") -> (before substring=w417:string, after substring=w416:string)  [unwired: 1 in, 2 out]
    n203 = case shown="\"idle\", Default" w417 {
      tunnel: w416 -> [_ _ _ _]
      tunnel: w415 -> [_ w480 w491 w499]
      tunnel: [_ TRUE _ _] -> w414
      tunnel: [0 _ -1 0] -> w412
      tunnel: [w446 w476 w490 w500] -> w411
      tunnel: w410 -> [w444 w476 w487 w507]
      tunnel: [w447 w475 refnum<k21> refnum ("task out") w501] -> w408
      tunnel: w407 -> [w445 w475 w488 _]
      tunnel: w406 -> [w448 _ _ _]
      tunnel: [w442 w473 w483 w496] -> w405
      tunnel: [w441 w474 w484 w497] -> w404
      tunnel: w403 -> [w439 w474 w484 w497]
      tunnel: w402 -> [w440 w473 w483 w496]
      tunnel: [w438 w472 w482 w495] -> w397
      tunnel: w401 -> [w437 w472 w482 w495]
      tunnel: w400 -> [_ w469 _ _]
      tunnel: [w426 w468 w481 w493] -> w399
      tunnel: w398 -> [w425 w468 w481 w493]
      frame "idle", Default {
        n204 = Dequeue Element(queue=w448, timeout in ms (-1)=0) -> (element=w443:dbl, timed out?=w427:bool)  [unwired: 1 in, 2 out]
        n205 = case shown="True" w427 {
          tunnel: w443 -> [w458 _]
          tunnel: [w458 w460] -> w436
          tunnel: [w458 w462] -> w442
          tunnel: [w452 w467] -> w441
          tunnel: w440 -> [w457 w462]
          tunnel: w439 -> [w456 w467]
          tunnel: [w453 w464] -> w438
          tunnel: w437 -> [_ w464]
          tunnel: [w452 w459] -> w426
          frame False {
            n206 = call <vilib>:"High Resolution Relative Seconds.vi"() -> ("relative seconds"=w452:dbl)
            n207 = Subtract(x=w458, y=w457) -> (x-y=w455:dbl)
            n208 = Subtract(x=w452, y=w456) -> (x-y=w454:dbl)
            n209 = Divide(x=w455, y=w454) -> (x/y=w453:dbl)
          }
          frame True {
            n210 = call <vilib>:"High Resolution Relative Seconds.vi"() -> ("relative seconds"=w459:dbl)
            n211 = Subtract(x=w459, y=w467) -> (x-y=w466:dbl)
            n212 = Multiply(x=w466, y=w464) -> (x*y=w465:dbl)
            n213 = Add(x=w462, y=w465) -> (x+y=w463:dbl)
            n214 = Select(t=w463, s="interpolate output", f=w462) -> (s? t:f=w460:dbl)
          }
        }
        n215 = local read "p1 [mm]"() -> (w434:dbl)
        n216 = local read "p2 [mm]"() -> (w435:dbl)
        n217 = Subtract(x=w436, y=w434) -> (x-y=w433:dbl)
        n218 = Subtract(x=w435, y=w434) -> (x-y=w432:dbl)
        n219 = Divide(x=w433, y=w432) -> (x/y=w431:dbl)
        n220 = Subtract(x=w426, y=w425) -> (x-y=w424:dbl)
        n221 = Multiply(x=w431, y=8.0) -> (x*y=w422:dbl)
        n222 = Reciprocal(x=w424) -> ()  [unwired: 1 out]
        n223 = Increment(x=w422) -> (x+1=w421:dbl)
        "x*y" <- w421
        n224 = In Range and Coerce(upper limit=10.0, x=w421, lower limit=0.0) -> (coerced(x)=w423:dbl)  [unwired: 1 out]
        "output voltage" <- w423
        n225 = case shown="True" "Enable?" {
          tunnel: w423 -> [_ w451]
          frame False {
          }
          frame True {
            "Waveform Chart" <- w451
          }
        }
        n226 = call-poly <vilib>:"DAQmx Write.vi"("task/channels in"=w445, "data"=w423, "error in"=w444) -> ("task out"=w447:refnum<k21>, "error out"=w446:errorcluster)  [unwired: 10 in, 1 out]
      }
      frame "close" {
        n227 = Dequeue Element(queue=w480) -> (queue out=w479:refnum<queue>, error out=w478:errorcluster)  [unwired: 2 in, 2 out]
        n228 = Unbundle By Name(w469) -> ("dev2_data"=w470:refnum<queue>)
        n229 = Release Queue(queue=w479, error in (no error)=w478) -> ()  [unwired: 1 in, 3 out]
        n230 = Flush Queue(queue=w470) -> (queue out=w471:refnum<queue>)  [unwired: 1 in, 2 out]
        n231 = Release Queue(queue=w471) -> ()  [unwired: 2 in, 3 out]
      }
      frame "release" {
        n232 = Dequeue Element(queue=w491) -> ()  [unwired: 2 in, 4 out]
        n233 = call <vilib>:"DAQmx Stop Task.vi"("task/channels in"=w488, "error in"=w487) -> ("task out"=w486:refnum<k21>, "error out"=w485:errorcluster)  [unwired: 12 in]
        n234 = call <vilib>:"DAQmx Clear Task.vi"("task in"=w486, "error in"=w485) -> ("error out"=w490:errorcluster)  [unwired: 13 in]
      }
      frame "initialize" {
        w504 = -1 items=["Default"=-1, "RSE"=10083, "Differential"=10106, "Pseudodifferential"=12529] ("output terminal configuration")
        n235 = Dequeue Element(queue=w499) -> ()  [unwired: 2 in, 4 out]
        n236 = call-poly <vilib>:"DAQmx Create Virtual Channel.vi"("maximum value"=10.0, "minimum value"=0.0, "output terminal configuration"=w504, "physical channels"="physical channels", "error in"=w507) -> ("task out"=w503:refnum<k21>, "error out"=w502:errorcluster)  [unwired: 9 in]
        n237 = call <vilib>:"DAQmx Start Task.vi"("task/channels in"=w503, "error in"=w502) -> ("task out"=w501:refnum<k21>, "error out"=w500:errorcluster)  [unwired: 12 in]
      }
    }
    "meas. velocity" <- w397
    "DAC error" <- w411
  }
